vi "DataSetDataToReferences.vi"(8 "error in (no error)":errorcluster, 11 "data event in":T1) -> (0 "error out":errorcluster, 3 "data event out":T1)   [LabVIEW 2017, in "FileManager.lvlib"]
uses:
  <vilib>/addons/InsightCM/Devices/Shared/Common/FileManager/FileManager.lvlib
  <vilib>/addons/InsightCM/Devices/Shared/Common/DataEvent/controls/Event.ctl
  <vilib>/addons/InsightCM/MessageBus/Base/controls/DataEvent.ctl
  <vilib>/addons/InsightCM/MessageBus/Base/controls/KeyValuePair.ctl
  <vilib>/addons/InsightCM/Devices/Shared/Common/DataEvent/controls/DataSet.ctl
  <vilib>/addons/InsightCM/MessageBus/Base/controls/DataSetMetadata.ctl
  <vilib>/addons/InsightCM/MessageBus/Base/controls/TrendPoint.ctl
  <vilib>/addons/InsightCM/MessageBus/Base/controls/TrendAlarmUpdate.ctl
  <vilib>/addons/InsightCM/MessageBus/Base/controls/TrendAlarmTransition.ctl
  <vilib>/addons/InsightCM/Devices/Shared/Common/DataEventCreator/DataEventCreator.lvlib
  <vilib>/addons/InsightCM/Devices/Shared/Common/DataEvent/DataEvent.lvlib
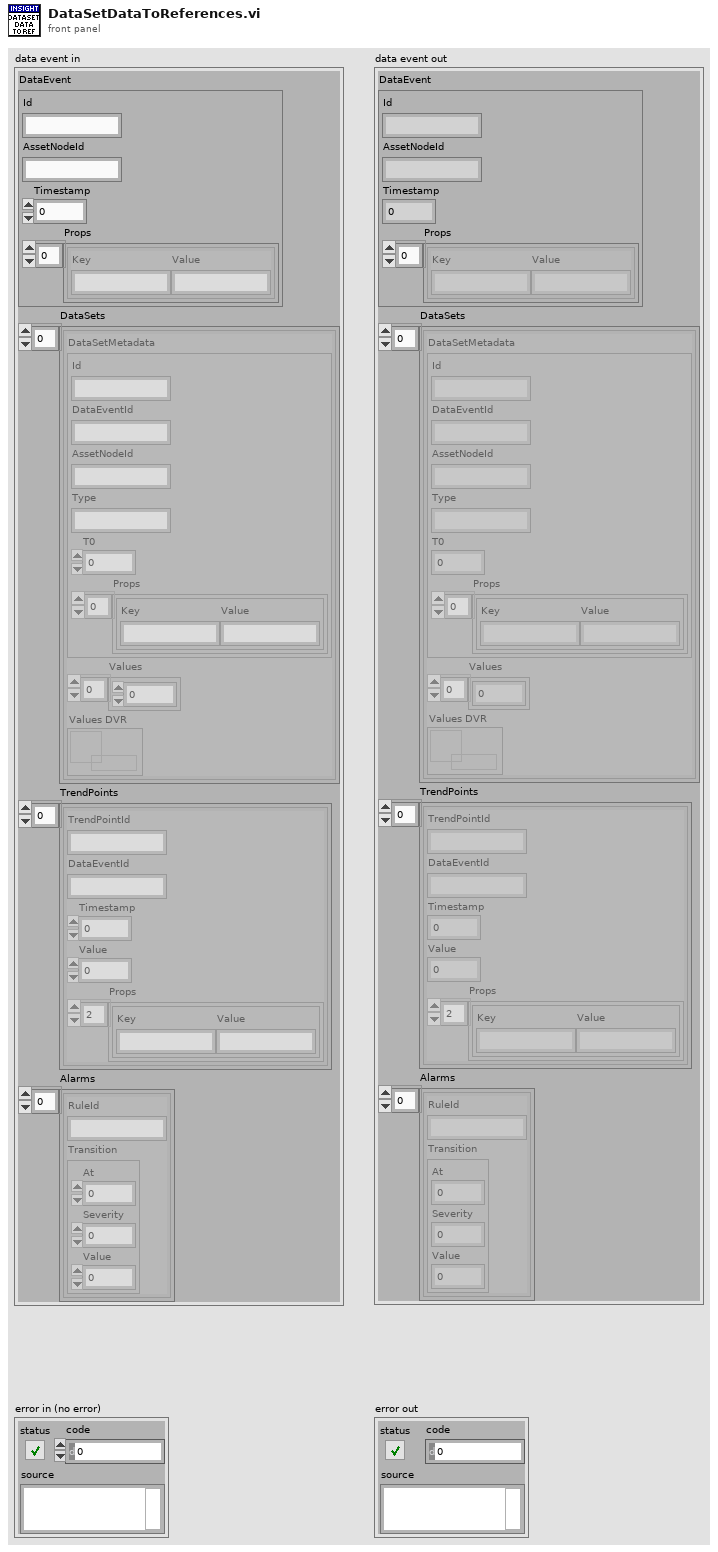
[diagram p1: front panel]
types:
  T1 = typedef "DataEvent.lvlib/Event.ctl" = cluster{"DataEvent":T2, "DataSets":T4[], "TrendPoints":T6[], "Alarms":T7[]}
  T2 = typedef "DataEvent.ctl" = cluster{"Id":string, "AssetNodeId":string, "Timestamp":i64, "Props":T3[]}
  T3 = typedef "KeyValuePair.ctl" = cluster{"Key":string, "Value":string}
  T4 = typedef "DataEvent.lvlib/DataSet.ctl" = cluster{"DataSetMetadata":T5, "Values":sgl[], "Values DVR":refnum<data-value>}
  T5 = typedef "DataSetMetadata.ctl" = cluster{"Id":string, "DataEventId":string, "AssetNodeId":string, "Type":string, "T0":i64, "Props":T3[]}
  T6 = typedef "TrendPoint.ctl" = cluster{"TrendPointId":string, "DataEventId":string, "Timestamp":i64, "Value":dbl, "Props":T3[]}
  T7 = typedef "TrendAlarmUpdate.ctl" = cluster{"RuleId":string, "Transition":T8}
  T8 = typedef "TrendAlarmTransition.ctl" = cluster{"At":i64, "Severity":i32, "Value":dbl}
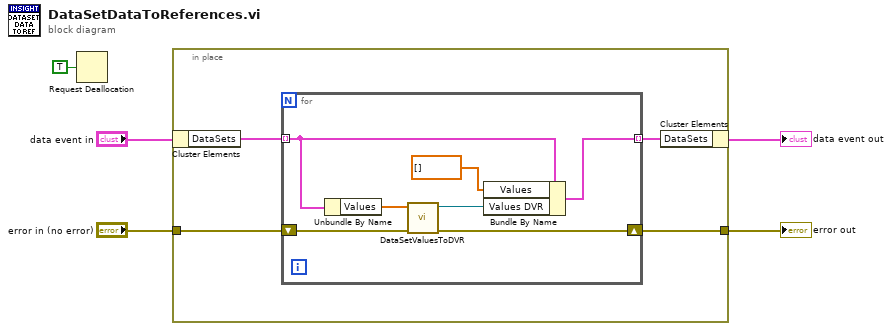
[diagram p0: block diagram]
diagram:
  n1 = Request Deallocation(TRUE ("flag")) -> ()
  n2 = in-place {
    in-place-border: "error in (no error)" -> [w7]
    in-place-border: [w6] -> w1
    n3 = in-place-cluster #1("data event in") -> ("DataSets"=w9:T4[])
    n4 = for {
      tunnel: w9 -> [w16] mode=indexing
      tunnel: [w10] -> w8 mode=indexing
      shift-right: [w11] -> w6
      shift-left: w7 -> [w12]
      n5 = Unbundle By Name(w16) -> ("Values"=w14:sgl[])
      n6 = call <vilib>:"DataSetValuesToDVR.vi"("error in (no error)"=w12, "dataset values"=w14) -> ("error out"=w11:errorcluster, "new dataset values dvr"=w13:refnum<data-value>)  [unwired: 8 in]
      n7 = Bundle By Name(cluster=w16, "Values"=sgl[] [], "Values DVR"=w13) -> (w10:T4)
    }
    n8 = in-place-cluster #1("DataSets"=w8) -> (→"data event out":T1)
  }
  "error out" <- w1
